vi "Library Open VI Ref Error Clarifier.vi"(0 "VI path":path, 11 "called VI error (no error)":errorcluster) -> (15 "error out":errorcluster)   [LabVIEW 2012]
doc: "This VI is designed to clarify errors generated by the Open VI Reference node by adding the path of the VI being opened to the error source."
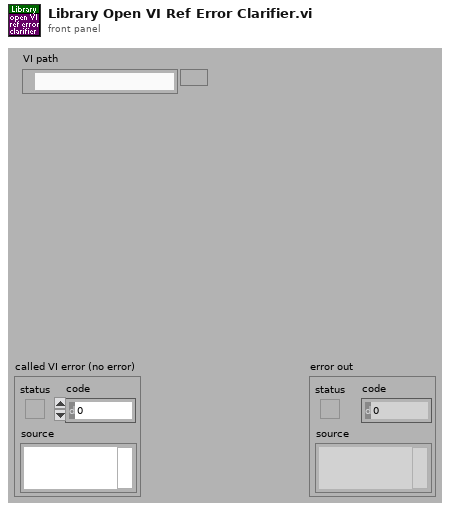
[diagram p1: front panel]
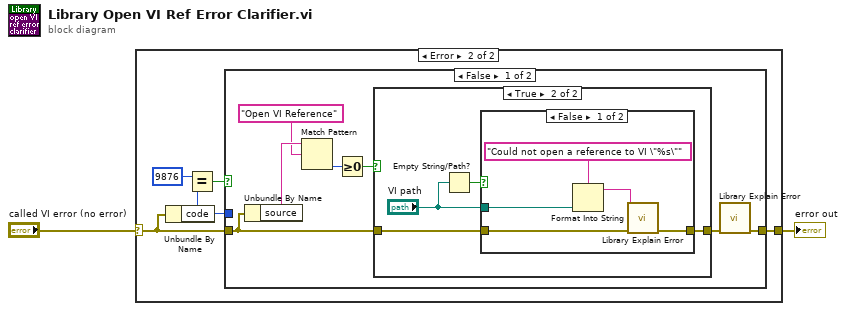
[diagram p0: block diagram]
diagram:
  n1 = case shown="Error" "called VI error (no error)" {
    selector: "called VI error (no error)" -> [w3 w4]
    tunnel: [w3 w8] -> w2
    frame No Error {
    }
    frame Error {
      n2 = Unbundle By Name(w4) -> ("code"=w7:i32)
      n3 = Equal?(x=9876, y=w7) -> (x = y?=w6:bool)
      n4 = case shown="False" w6 {
        tunnel: [w9 w27] -> w8
        tunnel: w7 -> [_ _]
        tunnel: w4 -> [w15 w27]
        frame False {
          n5 = Unbundle By Name(w15) -> ("source"=w14:string)
          n6 = Match Pattern(string=w14, regular expression="Open VI Reference" ("search string")) -> (offset past match=w11:i32)  [unwired: 1 in, 3 out]
          n7 = Greater Or Equal To 0?(x=w11) -> (x >= 0?=w12:bool)
          n8 = case shown="True" w12 {
            tunnel: [w16 w19] -> w10
            tunnel: w15 -> [w16 w20]
            frame False {
              # "An as yet not explained\nerror from some source\npreceeding the call to\n\"Open VI Reference\"."
            }
            frame True {
              n9 = Empty String/Path?(string/path="VI path") -> (empty?=w18:bool)
              n10 = case shown="False" w18 {
                tunnel: w20 -> [w23 w26]
                tunnel: [w21 w26] -> w19
                tunnel: "VI path" -> [w24 _]
                frame False {
                  n11 = Format Into String(format string="Could not open a reference to VI \"%s\"", w24) -> (resulting string=w22:string)  [unwired: 2 in, 1 out]
                  n12 = call "Library Explain Error.vi"("explanation prefix (none)"=w22, "error in (no error)"=w23) -> ("explained error"=w21:errorcluster)  [unwired: 13 in]
                }
                frame True {
                }
              }
            }
          }
          n13 = call "Library Explain Error.vi"("error in (no error)"=w10) -> ("explained error"=w9:errorcluster)  [unwired: 14 in]
        }
        frame True {
          # "Already an explained error."
        }
      }
    }
  }
  "error out" <- w2
